vi "InitializeEOMOutput.vi"(1 "Image Settings":T1={"Start Position (µm)"={"x"=0.0, "y"=0.0, "z"=0.0}, "End Position (µm)"={"x"=10.0, "y"=10.0, "z"=0.0}, "Image Resolution (nm/pixel)"={"x"=50.0, "y"=50.0, "z"=100.0}, "Image Size (µm)"={"x"=10.0, "y"=10.0, "z"=0.0}, "Image Size (pixel)"={"x"=50, "y"=50, "z"=0}, "Time Resolution\n(ms/pixel)"=7.0, "1st Axis"=0, "2nd Axis"=1, "Retrace"=FALSE, "Estimated Time"=""} {"2nd Axis" items=["x", "y", "z"]; "1st Axis" items=["x", "y", "z"]; "Time Resolution\n(ms/pixel)" format="%.2f"; "Image Resolution (nm/pixel)"."z" format="%.2f"; "Image Resolution (nm/pixel)"."y" format="%.2f"; "Image Resolution (nm/pixel)"."x" format="%.2f"; "Image Size (µm)"."z" format="%.2f"; "Image Size (µm)"."y" format="%.2f"; "Image Size (µm)"."x" format="%.2f"; "End Position (µm)"."z" format="%.2f"; "End Position (µm)"."y" format="%.2f"; "End Position (µm)"."x" format="%.2f"; "Start Position (µm)"."z" format="%.2f"; "Start Position (µm)"."y" format="%.2f"; "Start Position (µm)"."x" format="%.2f"}, 2 "EOM":u16(ring) items=["None", "Trace", "Retrace", "All"], 3 "Timing Info":T3 {"#s" format="%.2f"; "Fs" format="%.2f"}) -> (0 "Analog Output":T2)   [LabVIEW 2009]
uses:
  TimingInfo.ctt
  AnalogTrace.ctt
  ImageSettings.ctt
  <vilib>/Waveform/WDTOps.llb/WDT Append Waveforms DBL.vi
  <vilib>/measure/NI_MAPro.lvlib
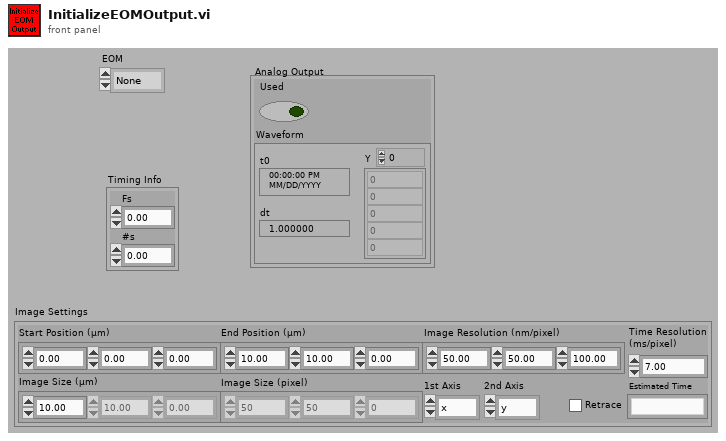
[diagram p1: front panel]
types:
  T1 = typedef "ImageSettings.ctt" = cluster{"Start Position (µm)":cluster{"x":dbl, "y":dbl, "z":dbl}, "End Position (µm)":cluster{"x":dbl, "y":dbl, "z":dbl}, "Image Resolution (nm/pixel)":cluster{"x":dbl, "y":dbl, "z":dbl}, "Image Size (µm)":cluster{"x":dbl, "y":dbl, "z":dbl}, "Image Size (pixel)":cluster{"x":u32, "y":u32, "z":u32}, "Time Resolution\n(ms/pixel)":dbl, "1st Axis":u16, "2nd Axis":u16, "Retrace":bool, "Estimated Time":string}
  T2 = typedef "AnalogTrace.ctt" = cluster{"Used":bool, "Waveform":waveform(dbl)}
  T3 = typedef "TimingInfo.ctt" = cluster{"Fs":dbl, "#s":dbl}
  T4 = typedef "EOMSettings.ctt" = cluster{"Output Channel":tag, "EOM Voltage":dbl, "Pixel per Polymode Cycle":u32, "Time per Polymode Cycle":dbl}
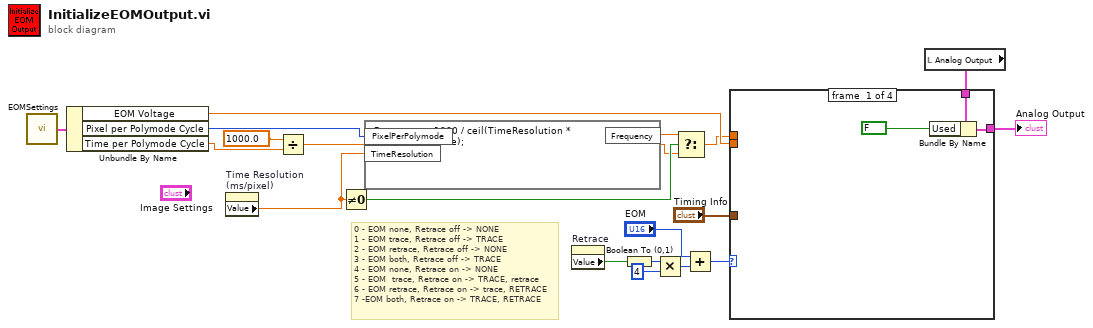
[diagram p0: block diagram]
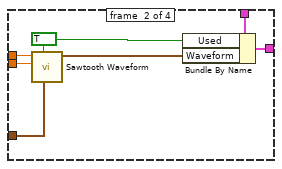
[diagram p2: hidden frame]
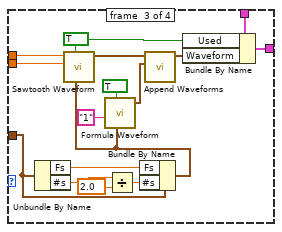
[diagram p3: hidden frame]
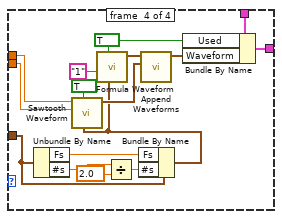
[diagram p4: hidden frame]
diagram:
  # "0 - EOM none, Retrace off -> NONE\n1 - EOM trace, Retrace off -> TRACE\n2 - EOM retrace, Retrace off -> NONE\n3 - EOM both, Retrace off -> TRACE\n4 - EOM none, Retrace on -> NONE\n5 - EOM  trace, Retrace on -> TRACE, retrace\n6 - EOM retrace, Retrace on -> trace, RETRACE\n7 -EOM both, Retrace on -> TRACE, RETRACE"
  n1 = call "EOMSettings.vi"() -> ("EOM Settings (output)"=w14:T4)  [unwired: 2 in]
  n2 = Unbundle By Name(w14) -> ("EOM Voltage"=w10:dbl, "Pixel per Polymode Cycle"=w8:u32, "Time per Polymode Cycle"=w3:dbl)
  n3 = property on="Time Resolution\n(ms/pixel)" class="Digital (strict)"() -> ("Value"=w6:dbl)  [unwired: 2 in, 2 out]
  n4 = Divide(x=1000.0 ("y"), y=w3) -> (x/y=w1:dbl)
  n5 = Not Equal To 0?(x=w6) -> (x != 0?=w7:bool)
  n6 = formula code="Frequency =1000 / ceil(TimeResolution * PixelPerPolymode);"("PixelPerPolymode"=w8, "TimeResolution"=w6) -> ("Frequency"=w5:dbl)
  n7 = property on="Retrace" class="Boolean (strict)"() -> ("Value"=w9:bool)  [unwired: 2 in, 2 out]
  n8 = Boolean To (0,1)(Boolean=w9) -> (0, 1=w19:i16)
  n9 = Multiply(x=w19, y=i16 4) -> (x*y=w17:i16)
  n10 = Select(t=w5, s=w7, f=w1) -> (s? t:f=w4:dbl)
  n11 = Add(x="EOM", y=w17) -> (x+y=w15:u16)
  n12 = local read "Analog Output"() -> (w12:T2)
  n13 = case shown="5" w15 {
    tunnel: w4 -> [_ w28 w44 w60]
    tunnel: w10 -> [_ w29 w45 w61]
    tunnel: "Timing Info" -> [_ w27 w35 w47]
    tunnel: w12 -> [w21 w24 w39 w59]
    tunnel: [w22 w23 w42 w58] -> w11
    frame #0 {
      n14 = Bundle By Name(cluster=w21, "Used"=FALSE) -> (w22:T2)
    }
    frame #1 {
      w26 = TRUE ("reset signal")
      n15 = call "Sawtooth Waveform.vi"("sampling info"=w27, "reset signal"=w26, "amplitude"=w29, "frequency"=w28) -> ("signal out"=w25:waveform(dbl))  [unwired: 6 in, 1 out]
      n16 = Bundle By Name(cluster=w24, "Used"=w26, "Waveform"=w25) -> (w23:T2)
    }
    frame #2 {
      w43 = TRUE ("reset signal")
      n17 = Unbundle By Name(w35) -> ("Fs"=w34:dbl, "#s"=w33:dbl)
      n18 = Divide(x=w33, y=2.0) -> (x/y=w31:dbl)
      n19 = Bundle By Name(cluster=w35, "Fs"=w34, "#s"=w31) -> (w30:T3)
      n20 = call "Sawtooth Waveform.vi"("sampling info"=w30, "reset signal"=w43, "amplitude"=w45, "frequency"=w44) -> ("signal out"=w38:waveform(dbl))  [unwired: 6 in, 1 out]
      n21 = call <vilib>:"Formula Waveform.vi"("sampling info"=w30, "reset signal"=TRUE, "formula"="1") -> ("signal out"=w37:waveform(dbl))  [unwired: 7 in, 1 out]
      n22 = call-poly <vilib>:"Append Waveforms.vi"("waveform B"=w37, "waveform A"=w38) -> ("waveform out"=w36:waveform(dbl))  [unwired: 8 in, 1 out]
      n23 = Bundle By Name(cluster=w39, "Used"=w43, "Waveform"=w36) -> (w42:T2)
    }
    frame #3 {
      w55 = TRUE ("reset signal")
      n24 = Unbundle By Name(w47) -> ("Fs"=w51:dbl, "#s"=w50:dbl)
      n25 = Divide(x=w50, y=2.0) -> (x/y=w48:dbl)
      n26 = Bundle By Name(cluster=w47, "Fs"=w51, "#s"=w48) -> (w46:T3)
      n27 = call "Sawtooth Waveform.vi"("sampling info"=w46, "reset signal"=TRUE, "amplitude"=w61, "frequency"=w60) -> ("signal out"=w53:waveform(dbl))  [unwired: 6 in, 1 out]
      n28 = call <vilib>:"Formula Waveform.vi"("sampling info"=w46, "reset signal"=w55, "formula"="1") -> ("signal out"=w54:waveform(dbl))  [unwired: 7 in, 1 out]
      n29 = call-poly <vilib>:"Append Waveforms.vi"("waveform B"=w53, "waveform A"=w54) -> ("waveform out"=w52:waveform(dbl))  [unwired: 8 in, 1 out]
      n30 = Bundle By Name(cluster=w59, "Used"=w55, "Waveform"=w52) -> (w58:T2)
    }
  }
  "Analog Output" <- w11
